vi "lee_EETT.vi"(8 "error in (no error)":errorcluster, 11 "Base de Datos in":refnum<class "Base de Datos.lvclass">) -> (0 "error out":errorcluster, 3 "Base de Datos out":refnum<class "Base de Datos.lvclass">)   [LabVIEW 2019, in "Base de Datos.lvclass"]
uses:
  Base de Datos.lvclass
  SQLiteConnector/SQLiteConnection.lvclass
panel:
  in  "Tipo Equipo":enum16{"Sonometro", "Calibrador", "Dosimetro"}(ring)
  out "result":string[][](array[string])
  out "query":string
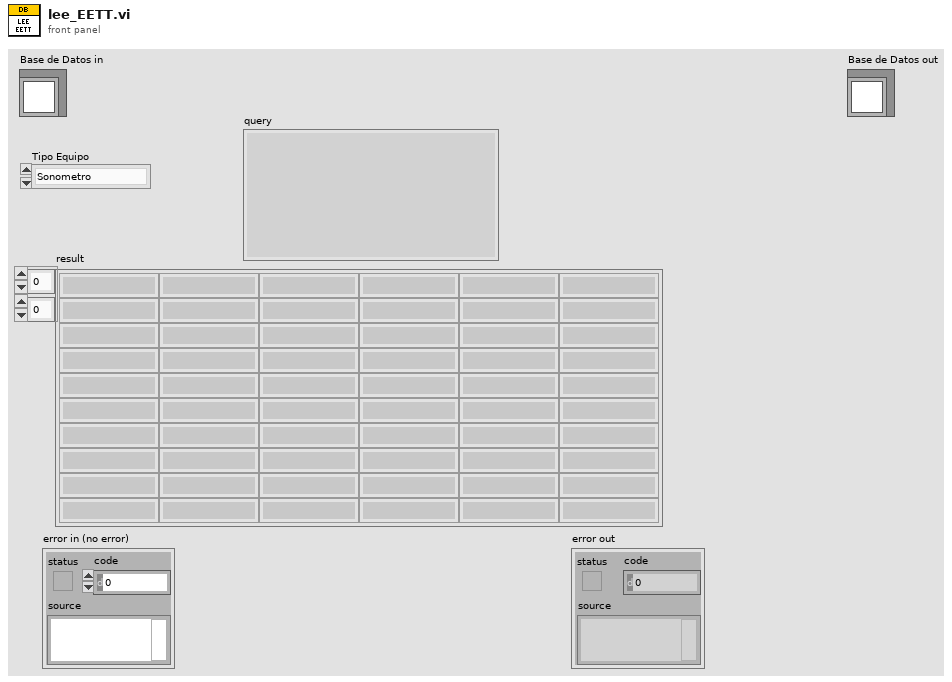
[diagram p1: front panel]
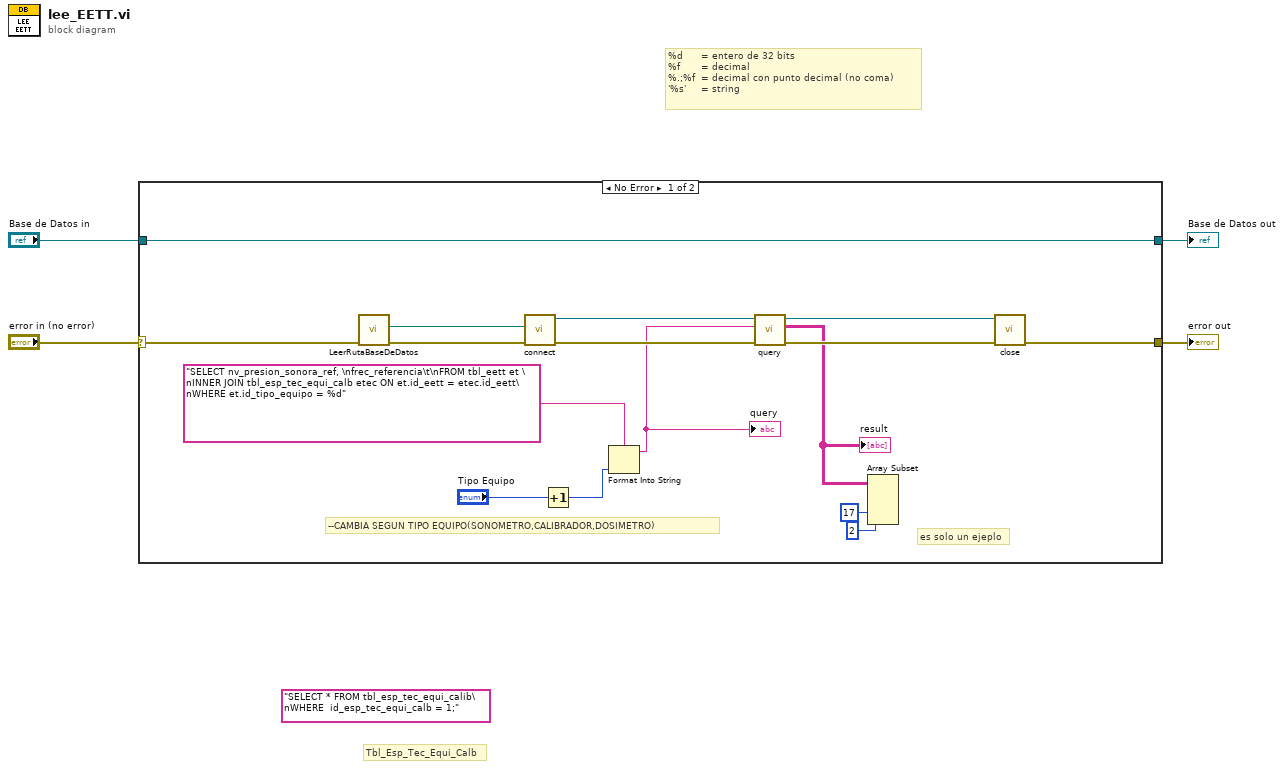
[diagram p0: block diagram]
diagram:
  (unwired) "SELECT * FROM tbl_esp_tec_equi_calib\nWHERE  id_esp_tec_equi_calb = 1;" ("format string")
  # "Tbl_Esp_Tec_Equi_Calb"
  # "%d      = entero de 32 bits\n%f       = decimal\n%.;%f  = decimal con punto decimal (no coma)\n'%s'     = string"
  n1 = case shown="No Error" "error in (no error)" {
    selector: "error in (no error)" -> [w13 w21]
    tunnel: [w19 w21] -> w4
    tunnel: "Base de Datos in" -> [w14 w22]
    tunnel: [w14 w22] -> w1
    frame No Error {
      # "--CAMBIA SEGUN TIPO EQUIPO(SONOMETRO,CALIBRADOR,DOSIMETRO)"
      # "es solo un ejeplo"
      n2 = call "LeerRutaBaseDeDatos.vi"("error in (no error)"=w13) -> ("error out"=w12:errorcluster, "Database Path"=w11:path)  [unwired: 9 in]
      n3 = call "connect.vi"("error in (no error)"=w12, "Database Path"=w11) -> ("error out"=w6:errorcluster, "object out"=w7:refnum<class "SQLiteConnection.lvclass">)  [unwired: 8 in]
      n4 = Increment(x="Tipo Equipo") -> (x+1=w9:enum16{"Sonometro", "Calibrador", "Dosimetro"})
      n5 = Format Into String(format string="SELECT nv_presion_sonora_ref, \nfrec_referencia\t\nFROM tbl_eett et \nINNER JOIN tbl_esp_tec_equi_calb etec ON et.id_eett = etec.id_eett\nWHERE et.id_tipo_equipo = %d", w9) -> (resulting string=w5:string)  [unwired: 2 in, 1 out]
      "query" <- w5
      n6 = call "query.vi"("error in (no error)"=w6, "SQL Statement"=w5, "object in"=w7) -> ("error out"=w20:errorcluster, "result"=w17:string[][], "object out"=w18:refnum<class "SQLiteConnection.lvclass">)  [unwired: 5 in, 1 out]
      "result" <- w17
      n7 = Array Subset(array=w17, index (col)=17 ("index"), length (col)=2 ("length")) -> ()  [unwired: 2 in, 1 out]
      n8 = call-dynamic "close.vi"("error in (no error)"=w20, "object in"=w18) -> ("error out"=w19:errorcluster)  [unwired: 8 in, 1 out]
    }
    frame Error {
    }
  }
  "error out" <- w4
  "Base de Datos out" <- w1
